vi "Teleop.vi"(10 "Match Info":T1={"Autonomous Elapsed Seconds"=0.0, "TeleOp Elapsed Seconds"=0.0, "Disabled Elapsed Seconds"=0.0, "Visited Autonomous"=FALSE, "Visited TeleOp"=FALSE, "Visited Disabled"=FALSE, "Autonomous Settings"={"Autonomous Style"=enum."Independent", "VI Refnum"=refnum}}, 11 "Call Context":T2) -> ()   [LabVIEW 2015]
doc: "This VI is called for each enabled TeleOp packet received from the DS. It is typically used to read from joysticks and other inputs and update I/O or setpoints for timed control loops. It should complete and return within 20 milliseconds or risk missing DS packets."
uses:
  <vilib>/Rock Robotics/WPI/DriverStation/WPI_DriverStationDerivedRobotMode.ctl
  <vilib>/Rock Robotics/WPI/DriverStation/WPI_DriverStationMatch Info.ctl
  Support Code/Team900-VIs/Logitech/F510/F510-X.vi
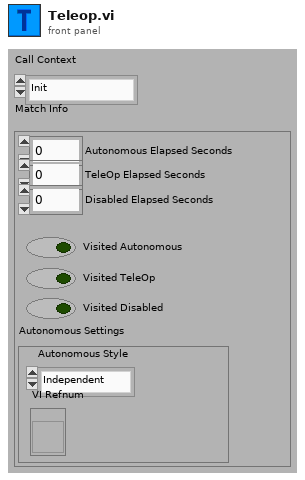
[diagram p1: front panel]
types:
  T1 = typedef "WPI_DriverStationMatch Info.ctl" = cluster{"Autonomous Elapsed Seconds":dbl, "TeleOp Elapsed Seconds":dbl, "Disabled Elapsed Seconds":dbl, "Visited Autonomous":bool, "Visited TeleOp":bool, "Visited Disabled":bool, "Autonomous Settings":cluster{"Autonomous Style":enum16{"Iterative", "Independent"}, "VI Refnum":refnum<vi>}}
  T2 = typedef "WPI_DriverStationDerivedRobotMode.ctl" = enum16{"Init", "Execute", "Stop"}
  T3 = cluster{"A":bool, "B":bool, "X":bool, "Y":bool, "LB":bool, "RB":bool, "Back":bool, "Start":bool, "LC":bool, "RC":bool, "LT":bool, "RT":bool}
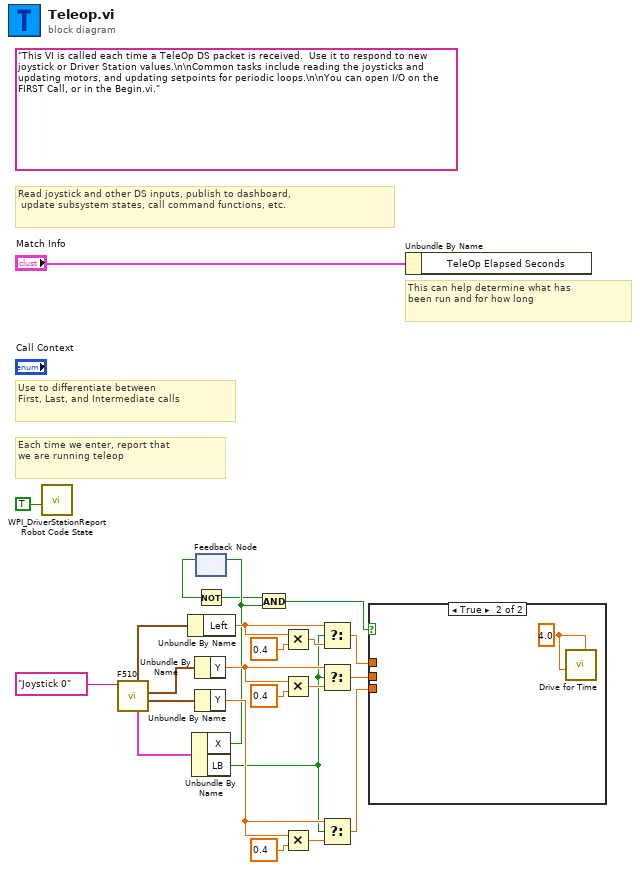
[diagram p0: block diagram]
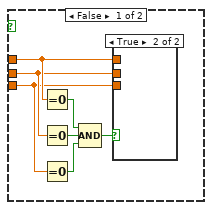
[diagram p2: hidden frame]
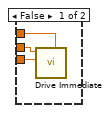
[diagram p3: hidden frame]
diagram:
  (unwired) "This VI is called each time a TeleOp DS packet is received.  Use it to respond to new joystick or Driver Station values.\n\nCommon tasks include reading the joysticks and updating motors, and updating setpoints for periodic loops.\n\nYou can open I/O on the FIRST Call, or in the Begin.vi."
  # "Read joystick and other DS inputs, publish to dashboard,\n update subsystem states, call command functions, etc."
  # "Each time we enter, report that\nwe are running teleop"
  # "Use to differentiate between\nFirst, Last, and Intermediate calls"
  # "This can help determine what has\nbeen run and for how long"
  n1 = call <vilib>:"WPI_DriverStationReport Robot Code State.vi"("TeleOp"=TRUE ("Autonomous")) -> ()  [unwired: 10 in, 1 out]
  n2 = call-poly "F510.vi"("refnum name"="Joystick 0") -> ("Right Stick"=w20:cluster{"X":dbl, "Y":dbl}, "Left Stick"=w21:cluster{"X":dbl, "Y":dbl}, "Buttons"=w18:T3, "Triggers"=w19:cluster{"Left":dbl, "Right":dbl})  [unwired: 4 in, 3 out]
  n3 = Unbundle By Name(w19) -> ("Left"=w8:dbl)
  n4 = Unbundle By Name(w18) -> ("X"=w4:bool, "LB"=w9:bool)
  n5 = Unbundle By Name(w21) -> ("Y"=w12:dbl)
  n6 = Unbundle By Name(w20) -> ("Y"=w16:dbl)
  n7 = feedback-in #1(w4) -> ()
  n8 = feedback #1() -> (w3:bool)  [unwired: 1 in]
  n9 = Not(x=w3) -> (.not. x?=w2:bool)
  n10 = And(x=w2, y=w4) -> (x .and. y?=w1:bool)
  n11 = Multiply(x=w8, y=0.4) -> (x*y=w11:dbl)
  n12 = Multiply(x=w12, y=0.4) -> (x*y=w14:dbl)
  n13 = Multiply(x=w16, y=0.4) -> (x*y=w17:dbl)
  n14 = Select(t=w8, s=w9, f=w11) -> (s? t:f=w5:dbl)
  n15 = Select(t=w12, s=w9, f=w14) -> (s? t:f=w6:dbl)
  n16 = Select(t=w16, s=w9, f=w17) -> (s? t:f=w7:dbl)
  n17 = case shown="True" w1 {
    tunnel: w7 -> [w26 _]
    tunnel: w6 -> [w27 _]
    tunnel: w5 -> [w28 _]
    frame False {
      n18 = Equal To 0?(x=w28) -> (x = 0?=w30:bool)
      n19 = Equal To 0?(x=w27) -> (x = 0?=w31:bool)
      n20 = Equal To 0?(x=w26) -> (x = 0?=w29:bool)
      n21 = Compound Arithmetic op=AND(w30, w31, w29) -> (w25:bool)
      n22 = case shown="True" w25 {
        tunnel: w27 -> [w34 _]
        tunnel: w28 -> [w33 _]
        tunnel: w26 -> [w32 _]
        frame False {
          n23 = call "Drive Immediate.vi"("Straight Setpoint"=w33, "Right Setpoint"=w32, "Left Setpoint"=w34) -> ()  [unwired: 8 in, 1 out]
        }
        frame True {
        }
      }
    }
    frame True {
      w35 = 4.0
      n24 = call "Drive for Time.vi"("Straight Setpoint"=w35, "Seconds"=w35) -> ()  [unwired: 8 in, 2 out]
    }
  }
  n25 = Unbundle By Name("Match Info") -> ()  [unwired: 1 out]
